vi "Rotation2d_CreateAngle.vi"(11 "Angle (Radians)":dbl) -> (3 "ROTATION":T1 {"SIN" format="%13.4f"; "COS" format="%13.4f"; "VALUE" format="%13.4f"})   [LabVIEW 2020, in "Swerve_Odometry_SEN.lvlib"]
doc: "Constructs a Rotation2d with the given radian value. The x and y don't have to be normalized.\n\nParmeters:\n - value - The value of the angle in radians.\n\nReturns\n - rotation data structure"
uses:
  Swerve_Odometry_SEN.lvlib
  Cluster_ROTATION2D.ctl
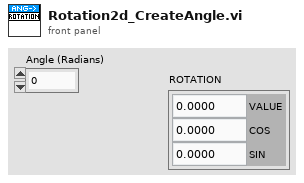
[diagram p1: front panel]
types:
  T1 = typedef "Swerve_Odometry_SEN.lvlib/Cluster_ROTATION2D.ctl" = cluster{"VALUE":dbl, "COS":dbl, "SIN":dbl}
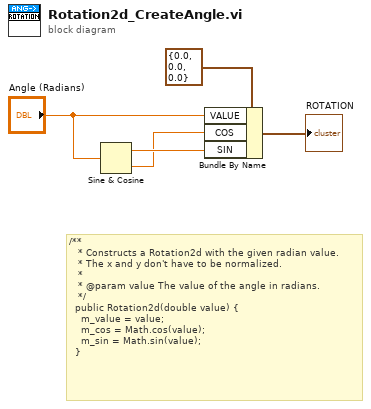
[diagram p0: block diagram]
diagram:
  # "/**\n   * Constructs a Rotation2d with the given radian value.\n   * The x and y don't have to be normalized.\n   *\n   * @param value The value of the angle in radians.\n   */\n  public Rotation2d(double value) {\n    m_value = value;\n    m_cos = Math.cos(value);\n    m_sin = Math.sin(value);\n  }"
  n1 = Sine & Cosine(0:"Angle (Radians)") -> (1:w3:dbl, 2:w2:dbl)
  n2 = Bundle By Name(cluster=T1 {"VALUE"=0.0, "COS"=0.0, "SIN"=0.0} ("ROTATION"), "VALUE"="Angle (Radians)", "COS"=w2, "SIN"=w3) -> (→"ROTATION":T1)
